vi "SMTP using LabVIEW.vi"   [LabVIEW 2025]
uses:
  <vilib>/smtpClient/LabVIEWSMTPClient.lvlib
  <vilib>/smtpClient/Set Message Text.vi
types:
  T1 = typedef "LabVIEWSMTPClient.lvlib/SmtpClientHandle.ctl" = refnum<k1>
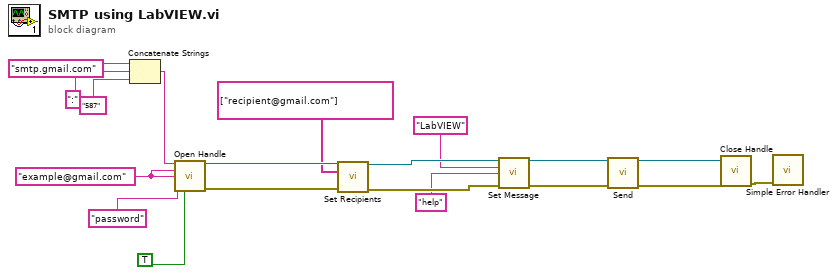
[diagram p0: block diagram]
diagram:
  w6 = "example@gmail.com" ("username")
  n1 = Concatenate Strings("smtp.gmail.com" ("string"), ":" ("string"), "587" ("string")) -> (w2:string)
  n2 = call <vilib>:"Open Handle.vi"("server address"=w2, "from"=w6, "username"=w6, "password"="password", "use TLS (false)"=TRUE) -> ("handle out"=w14:T1, "error out"=w19:errorcluster)  [unwired: 9 in]
  n3 = call <vilib>:"Set Recipients.vi"("handle in"=w14, "to"=string[] ["recipient@gmail.com"], "error in (no error)"=w19) -> ("handle out"=w13:T1, "error out"=w18:errorcluster)  [unwired: 11 in]
  n4 = call-poly <vilib>:"Set Message.vi"("handle in"=w13, "subject"="LabVIEW", "plain text message"="help", "error in (no error)"=w18) -> ("handle out"=w12:T1, "error out"=w17:errorcluster)  [unwired: 10 in]
  n5 = call <vilib>:"Send.vi"("handle in"=w12, "error in (no error)"=w17) -> ("handle out"=w11:T1, "error out"=w16:errorcluster)  [unwired: 11 in, 1 out]
  n6 = call <vilib>:"Close Handle.vi"("handle in"=w11, "error in (no error)"=w16) -> ("error out"=w15:errorcluster)  [unwired: 12 in, 1 out]
  n7 = call <vilib>:"Simple Error Handler.vi"("error in (no error)"=w15) -> ()  [unwired: 4 in, 5 out]
